vi "labview2tikz_WaveformGraph_Double.vi"(8 "error in (no error)":errorcluster, 10 "file (use dialog)":path, 11 "Waveform Graph":refnum<vi>) -> (0 "error out":errorcluster, 3 "result string":string)   [LabVIEW 2012]
uses:
  pgfPlotPlot_tdef.ctl
  <vilib>/Waveform/WDTOps.llb/WDT Get Waveform Time Array DBL.vi
  pgfPlotAxis_tdef.ctl
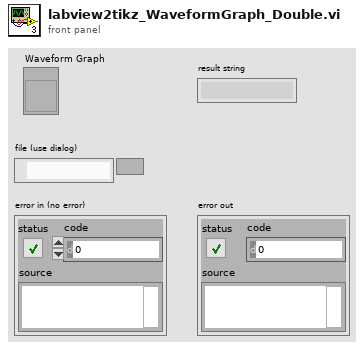
[diagram p1: front panel]
types:
  T1 = typedef "pgfPlotAxis_tdef.ctl" = cluster{"xmin":dbl, "xmax":dbl, "ymin":dbl, "ymax":dbl, "xLabel":string, "yLabel":string}
  T2 = typedef "pgfPlotPlot_tdef.ctl" = cluster{"LineStyle":u8, "LineWidth":u8, "PlotColor":u32, "Marker":u8, "PlotName":string, "x values":dbl[], "y values":dbl[]}
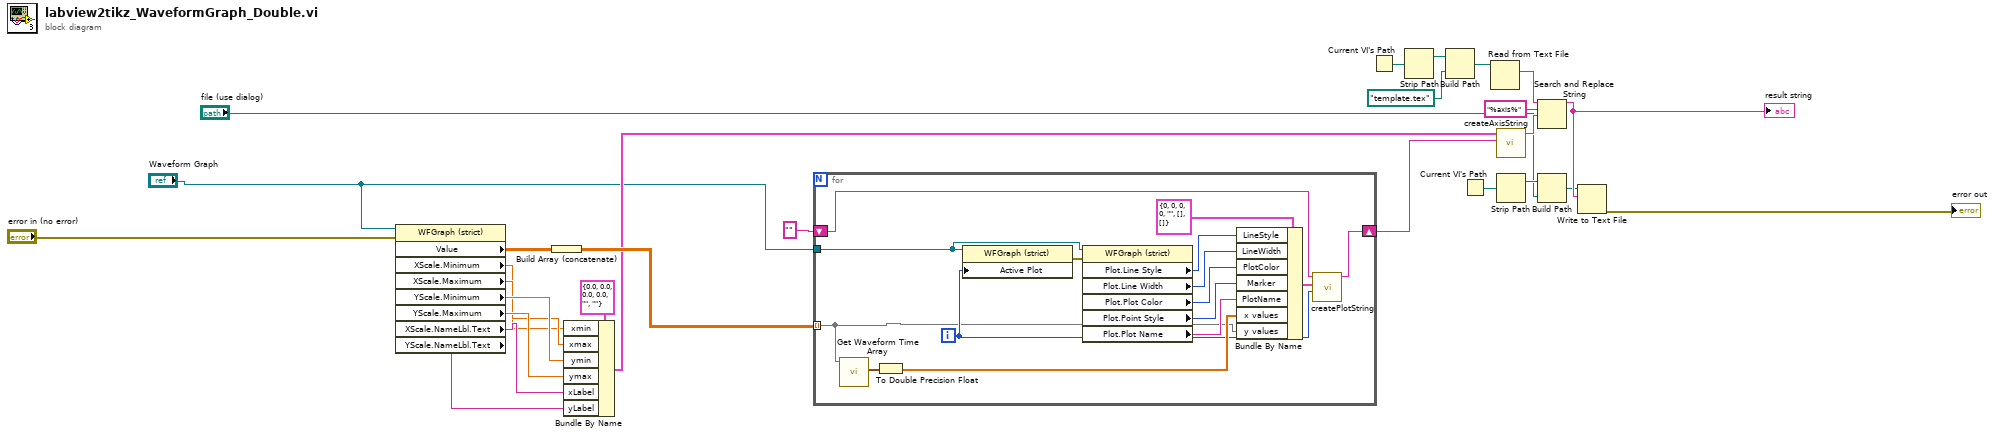
[diagram p0: block diagram]
diagram:
  n1 = property class="WFGraph (strict)"(reference="Waveform Graph", error in="error in (no error)") -> ("Value"=w10:dbl[][], "XScale.Minimum"=w14:dbl, "XScale.Maximum"=w15:dbl, "YScale.Minimum"=w16:dbl, "YScale.Maximum"=w17:dbl, "XScale.NameLbl.Text"=w18:string, "YScale.NameLbl.Text"=w19:string)  [unwired: 2 out]
  n2 = Build Array (concatenate)(w10) -> (w27:dbl[][])
  n3 = Bundle By Name(cluster=T1 {"xmin"=0.0, "xmax"=0.0, "ymin"=0.0, "ymax"=0.0, "xLabel"="", "yLabel"=""} ("Input"), "xmin"=w14, "xmax"=w15, "ymin"=w16, "ymax"=w17, "xLabel"=w18, "yLabel"=w19) -> (w20:T1)
  n4 = for {
    tunnel: "Waveform Graph" -> [w42]
    tunnel: w27 -> [w28] mode=indexing
    shift-right: [w39] -> w23
    shift-left: "" -> [w30]
    i -> [w29]
    n5 = call-poly <vilib>:"Get Waveform Time Array.vi"("waveform in"=w28) -> ("X array"=w41:timestamp[])  [unwired: 9 in, 1 out]
    n6 = To Double Precision Float(number=w41) -> (double precision float=w31:dbl[])
    n7 = property class="WFGraph (strict)"(reference=w42, "Active Plot"=w29) -> (error out=w40:errorcluster)  [unwired: 1 in, 1 out]
    n8 = property class="WFGraph (strict)"(reference=w42, error in=w40) -> ("Plot.Line Style"=w37:u8, "Plot.Line Width"=w36:u8, "Plot.Plot Color"=w32:u32, "Plot.Point Style"=w35:u8, "Plot.Plot Name"=w34:string)  [unwired: 2 out]
    n9 = Bundle By Name(cluster=T2 {"LineStyle"=0, "LineWidth"=0, "PlotColor"=0, "Marker"=0, "PlotName"="", "x values"=[], "y values"=[]}, "LineStyle"=w37, "LineWidth"=w36, "PlotColor"=w32, "Marker"=w35, "PlotName"=w34, "x values"=w31, "y values"=w28) -> (w33:T2)
    n10 = call "createPlotString.vi"("current plot number"=w29, "Plot Data"=w33, "plot string in"=w30) -> ("plot string out"=w39:string)  [unwired: 8 in]
  }
  n11 = Current VI's Path() -> (path=w2:path)
  n12 = Strip Path(path=w2) -> (stripped path=w3:path)  [unwired: 1 out]
  n13 = Build Path(base path=w3, name or relative path=path "template.tex" ("file (use dialog)")) -> (appended path=w5:path)
  n14 = Current VI's Path() -> (path=w8:path)
  n15 = Read from Text File(file (use dialog)=w5) -> (text=w12:string)  [unwired: 3 in, 3 out]
  n16 = call "createAxisString.vi"("PlotsString"=w23, "Input Data"=w20) -> ("AxisString"=w22:string)  [unwired: 9 in]
  n17 = Strip Path(path=w8) -> (stripped path=w7:path)  [unwired: 1 out]
  n18 = Search and Replace String(input string=w12, search string="%axis%", replace string=w22) -> (result string=w24:string)  [unwired: 5 in, 3 out]
  "result string" <- w24
  n19 = Build Path(base path=w7, name or relative path="file (use dialog)") -> (appended path=w9:path)
  n20 = Write to Text File(file (use dialog)=w9, text=w24) -> (error out=→"error out":errorcluster)  [unwired: 2 in, 2 out]
